vi "LWXPS_PositionerCorrectorPIPositionSet.vi"(0 "Positioner Name":string, 1 "XPS Reference IN":refnum<k24>, 5 "Closed Loop Status":bool, 7 "Proportional Gain":dbl, 9 "Integral Gain":dbl, 11 "Integration Time":dbl, 12 "LabVIEW error IN":errorcluster) -> (4 "XPS Reference OUT":refnum<k24>, 6 "Returned error code":i32, 8 "XPS Error String":string, 15 "LabVIEW error OUT":errorcluster)   [LabVIEW 2014]
uses:
  D:/XPSQ8_LabView_Library/Development/Source/Dll/Newport.XPS.CommandInterface.dll
  Dll/Newport.XPS.CommandInterface.dll
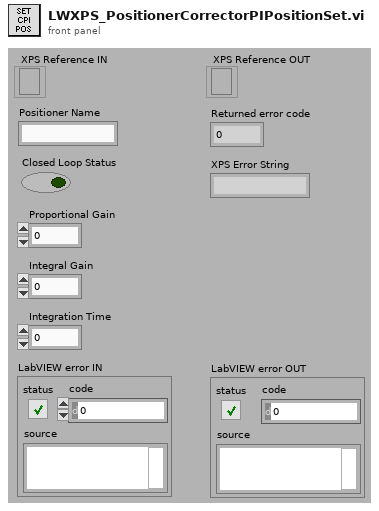
[diagram p1: front panel]
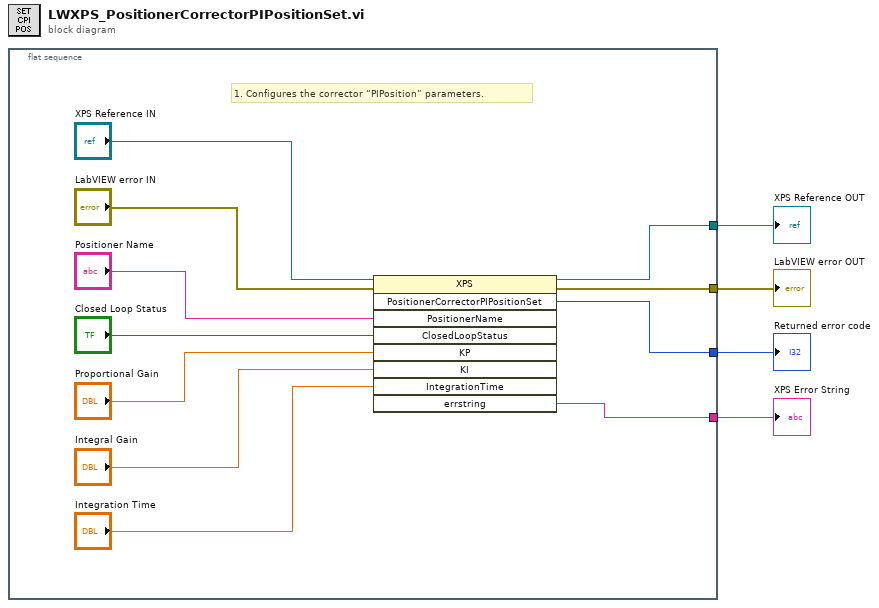
[diagram p0: block diagram]
diagram:
  n1 = flat-sequence {
    tunnel: [w11] -> w4
    tunnel: [w10] -> w3
    tunnel: [w12] -> w2
    tunnel: [w7] -> w1
    frame #0 {
      # "1. Configures the corrector “PIPosition” parameters."
      n2 = invoke class="XPS" method="PositionerCorrectorPIPositionSet"(reference="XPS Reference IN", error in="LabVIEW error IN", "PositionerName"="Positioner Name", "ClosedLoopStatus"="Closed Loop Status", "KP"="Proportional Gain", "KI"="Integral Gain", "IntegrationTime"="Integration Time") -> (reference out=w11:refnum<k24>, error out=w10:errorcluster, "PositionerCorrectorPIPositionSet"=w12:i32, "errstring"=w7:string)  [unwired: 2 in, 5 out]
    }
  }
  "XPS Error String" <- w1
  "XPS Reference OUT" <- w4
  "LabVIEW error OUT" <- w3
  "Returned error code" <- w2
